vi "TLC Geometry - Batch Alignment.vi"() -> ()   [LabVIEW 2023]
doc: "This example shows how to use the Batch Alignment VIs to align a list of controls."
uses:
  <vilib>/numeric/Random Number (Range) U64.vi
  <vilib>/numeric/sub_Random U32.vi
panel:
  in  "distributeVerticalCenters":bool
  in  "distributeHorizontalCenters":bool
  in  "alignHorizontalCenters":bool
  in  "alignVerticalCenters":bool
  in  "alignBottom":bool
  in  "alignTop":bool
  in  "useControlBodyOnly":bool=TRUE caption="Use Ctrl Body Only\n(=ignore labels \n& captions)"
  in  "stop":bool
  in  "alignRight":bool
  in  "alignLeft":bool
  in  "shuffle":bool
  in  "control 3":string
  in  "control 2":bool
  in  "control 1":string
  in  "control 0":dbl
  # "Instruction:\n1. Press Shuffle button to place the target objects randomly.\n2. Press the Alignment button you prefer."
  # "Batch alignment"
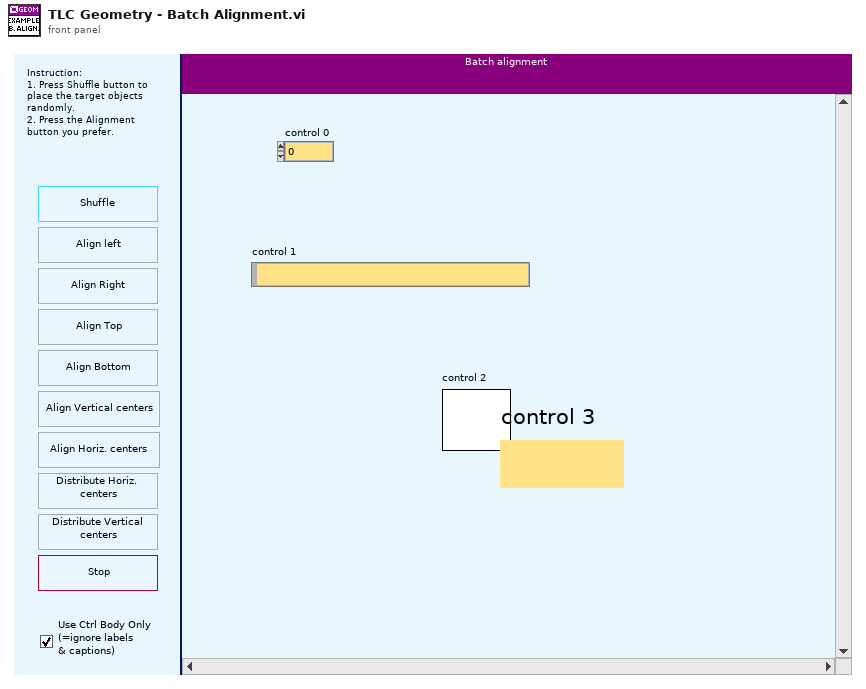
[diagram p1: front panel]
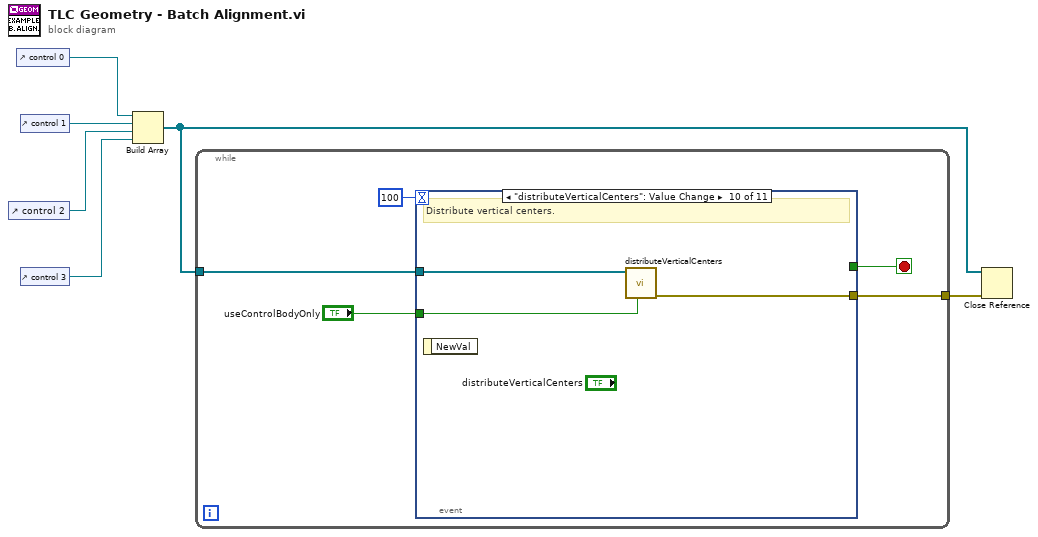
[diagram p0: block diagram]
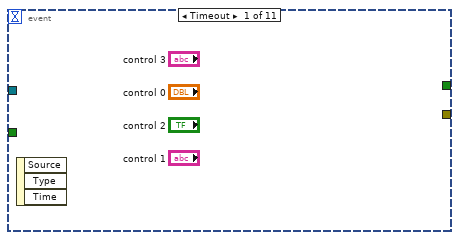
[diagram p2: hidden frame]
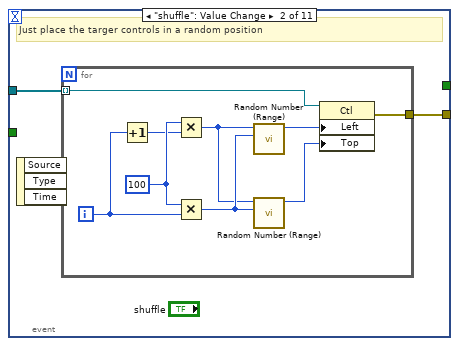
[diagram p3: hidden frame]
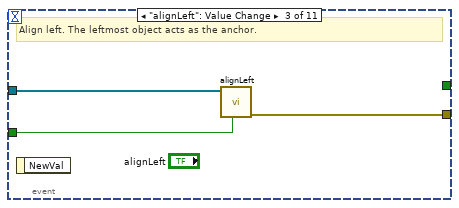
[diagram p4: hidden frame]
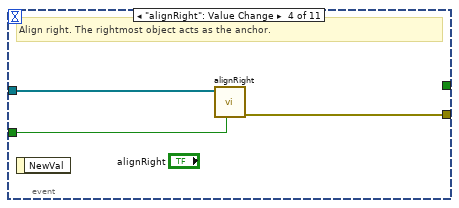
[diagram p5: hidden frame]
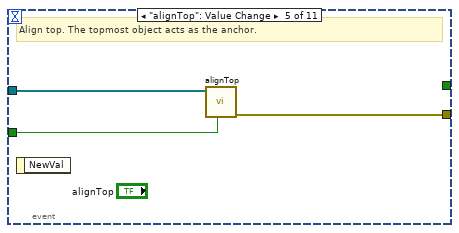
[diagram p6: hidden frame]
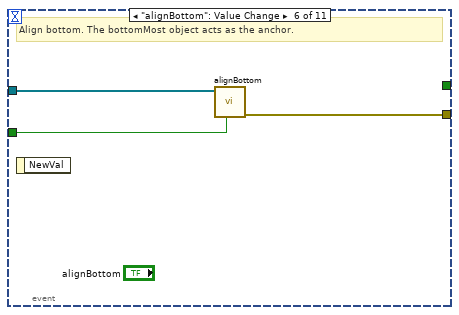
[diagram p7: hidden frame]
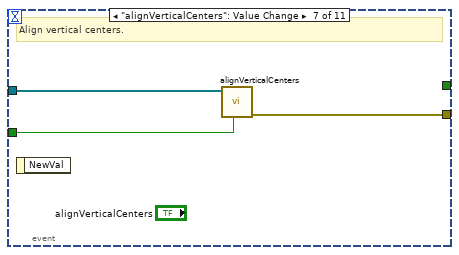
[diagram p8: hidden frame]
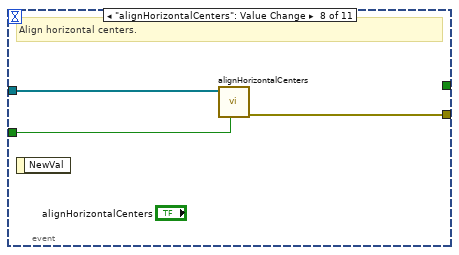
[diagram p9: hidden frame]
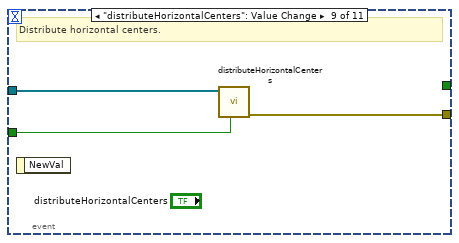
[diagram p10: hidden frame]
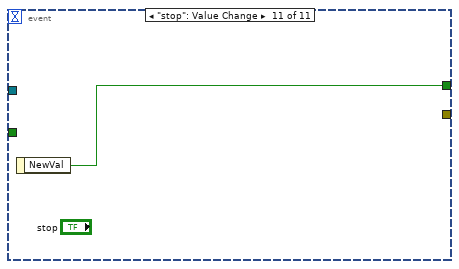
[diagram p11: hidden frame]
diagram:
  n1 = control-ref of="control 2"() -> (w5:refnum<vi>)
  n2 = control-ref of="control 0"() -> (w1:refnum<vi>)
  n3 = control-ref of="control 1"() -> (w6:refnum<vi>)
  n4 = control-ref of="control 3"() -> (w4:refnum<vi>)
  n5 = Build Array(w1, w6, w5, w4) -> (w3:refnum<vi>[])
  n6 = while {
    tunnel: w3 -> [w10]
    tunnel: [w9] -> w2
    stop <- w11 stop-if-true
    n7 = event shown="[9] \"distributeVerticalCenters\": Value Change" {
      selector: _ -> [_ _ _ _ _ _ _ _ _ _ _]
      dyn-events: _ -> [_ _ _ _ _ _ _ _ _ _ _]
      timeout: 100 -> [_ _ _ _ _ _ _ _ _ _ _]
      tunnel: [_ _ _ _ _ _ _ _ _ _ w47] -> w11
      tunnel: w10 -> [_ w13 w25 w28 w31 w34 w37 w40 w43 w46 _]
      tunnel: [_ w12 w23 w26 w29 w32 w35 w38 w41 w44 _] -> w9
      tunnel: "useControlBodyOnly" -> [_ _ w24 w27 w30 w33 w36 w39 w42 w45 _]
      event Timeout {
        n8 = event-data() -> ()  [unwired: 1 in, 3 out]
      }
      event "shuffle": Value Change {
        # "Just place the targer controls in a random position"
        n9 = event-data() -> ()  [unwired: 1 in, 3 out]
        n10 = for {
          tunnel: w13 -> [w22] mode=indexing
          tunnel: [w19] -> w12
          i -> [w18]
          w17 = u64 100 ("upper bound (100)")
          n11 = Increment(x=w18) -> (x+1=w15:i32)
          n12 = Multiply(x=w17, y=w15) -> (x*y=w14:u64)
          n13 = Multiply(x=w17, y=w18) -> (x*y=w16:u64)
          n14 = call-poly <vilib>:"Random Number (Range).vi"("lower bound (0)"=w16, "upper bound (100)"=w14) -> ("number"=w21:u64)  [unwired: 9 in]
          n15 = call-poly <vilib>:"Random Number (Range).vi"("lower bound (0)"=w16, "upper bound (100)"=w14) -> ("number"=w20:u64)  [unwired: 9 in]
          n16 = property class="Ctl"(reference=w22, "Left"=w21, "Top"=w20) -> (error out=w19:errorcluster)  [unwired: 1 in, 1 out]
        }
      }
      event "alignLeft": Value Change {
        # "Align left. The leftmost object acts as the anchor."
        n17 = event-data() -> ()  [unwired: 1 in, 1 out]
        n18 = call "alignLeft.vi"("useControlBodyOnly"=w24, "refs"=w25) -> ("error out"=w23:errorcluster)  [unwired: 8 in, 1 out]
      }
      event "alignRight": Value Change {
        # "Align right. The rightmost object acts as the anchor."
        n19 = event-data() -> ()  [unwired: 1 in, 1 out]
        n20 = call "alignRight.vi"("useControlBodyOnly"=w27, "refs"=w28) -> ("error out"=w26:errorcluster)  [unwired: 8 in, 1 out]
      }
      event "alignTop": Value Change {
        # "Align top. The topmost object acts as the anchor."
        n21 = event-data() -> ()  [unwired: 1 in, 1 out]
        n22 = call "alignTop.vi"("useControlBodyOnly"=w30, "refs"=w31) -> ("error out"=w29:errorcluster)  [unwired: 8 in, 1 out]
      }
      event "alignBottom": Value Change {
        # "Align bottom. The bottomMost object acts as the anchor."
        n23 = event-data() -> ()  [unwired: 1 in, 1 out]
        n24 = call "alignBottom.vi"("useControlBodyOnly"=w33, "refs"=w34) -> ("error out"=w32:errorcluster)  [unwired: 8 in, 1 out]
      }
      event "alignVerticalCenters": Value Change {
        # "Align vertical centers."
        n25 = event-data() -> ()  [unwired: 1 in, 1 out]
        n26 = call "alignVerticalCenters.vi"("useControlBodyOnly"=w36, "refs"=w37) -> ("error out"=w35:errorcluster)  [unwired: 8 in, 1 out]
      }
      event "alignHorizontalCenters": Value Change {
        # "Align horizontal centers."
        n27 = event-data() -> ()  [unwired: 1 in, 1 out]
        n28 = call "alignHorizontalCenters.vi"("useControlBodyOnly"=w39, "refs"=w40) -> ("error out"=w38:errorcluster)  [unwired: 8 in, 1 out]
      }
      event "distributeHorizontalCenters": Value Change {
        # "Distribute horizontal centers."
        n29 = event-data() -> ()  [unwired: 1 in, 1 out]
        n30 = call "distributeHorizontalCenters.vi"("useControlBodyOnly"=w42, "refs"=w43) -> ("error out"=w41:errorcluster)  [unwired: 8 in, 1 out]
      }
      event "distributeVerticalCenters": Value Change {
        # "Distribute vertical centers."
        n31 = event-data() -> ()  [unwired: 1 in, 1 out]
        n32 = call "distributeVerticalCenters.vi"("useControlBodyOnly"=w45, "refs"=w46) -> ("error out"=w44:errorcluster)  [unwired: 8 in, 1 out]
      }
      event "stop": Value Change {
        n33 = event-data() -> ("NewVal"=w47:bool)  [unwired: 1 in]
      }
    }
  }
  n34 = Close Reference(reference=w3, error in (no error)=w2) -> ()  [unwired: 1 out]
